vi "Write Methods.vi"(8 "error in (no error)":errorcluster, 10 "Methods":refnum<class "CS++Method.lvclass">[](array[class]), 11 "CS++Actor in":refnum<class "CS++Actor.lvclass">) -> (0 "error out":errorcluster, 3 "CS++Actor out":refnum<class "CS++Actor.lvclass">)   [LabVIEW 2014, in "CS++Actor.lvlib" / "CS++Actor.lvclass"]
uses:
  CS++Actor.lvclass
  CSPP_Method/CS++Method.lvclass
  CS++Actor.lvclass/CS++Actor.ctl
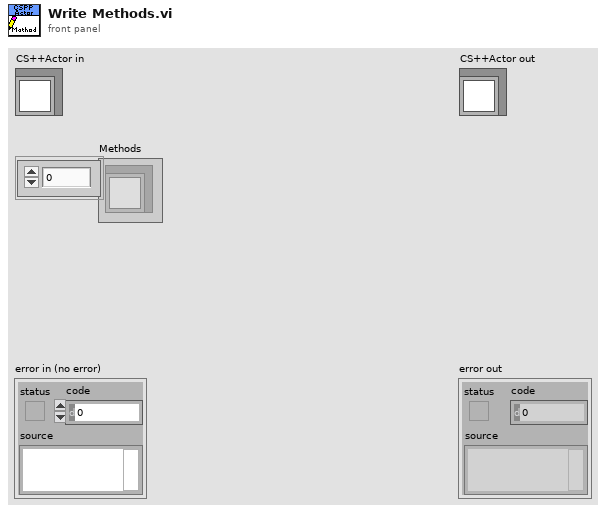
[diagram p1: front panel]
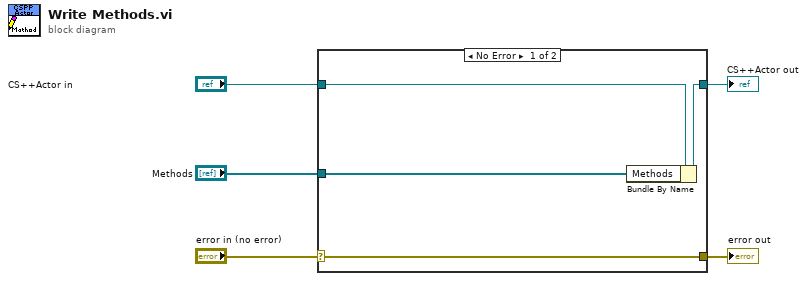
[diagram p0: block diagram]
diagram:
  n1 = case shown="No Error" "error in (no error)" {
    selector: "error in (no error)" -> [w9 w10]
    tunnel: [w9 w10] -> w4
    tunnel: [w7 w11] -> w2
    tunnel: "CS++Actor in" -> [w8 w11]
    tunnel: "Methods" -> [w6 _]
    frame No Error {
      n2 = Bundle By Name(cluster=w8, "Methods"=w6) -> (w7:refnum<class "CS++Actor.lvclass">)
    }
    frame Error {
    }
  }
  "error out" <- w4
  "CS++Actor out" <- w2
